vi "RVHR - File Selection.vi"(8 "error in":errorcluster) -> (0 "error out":errorcluster, 2 "cancelled?":bool caption="cancelled", 3 "RVHR path":path caption="selected path")   [LabVIEW 2024]
uses:
  Controls/Device_Type.ctl
  Controls/Language.ctl
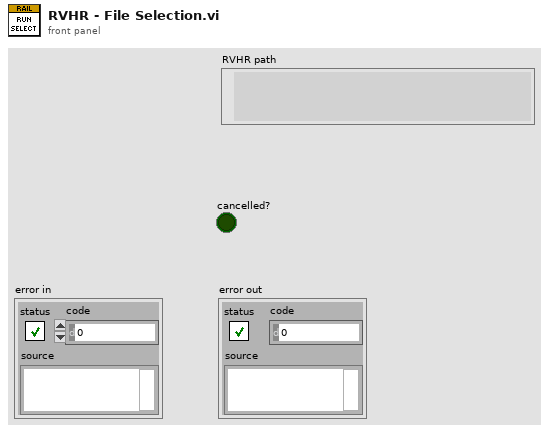
[diagram p1: front panel]
types:
  T1 = typedef "Device_Type.ctl" = enum16{"CAT", "Bi-CAT", "YRCA", "RCA", "RV-HR", "TV-HR"}
  T2 = typedef "Language.ctl" = enum16{"English", "Chinese", "German"}
  T3 = cluster{"Run Start":dbl, "Run End":dbl, "Date":timestamp}
  T4 = typedef "RVHR - Local Data.ctl" = cluster{"Main Filtered Data":dbl[][][], "Main Dist Data":dbl[], "Comp Filtered Data":dbl[][][], "Comp Dist Data":dbl[], "Image":u16, "Total Images":u16, "Main Test Cluster":T5, "Main Dates-Times":cluster{"Start Date":string, "Start Time":string, "Finish Time":string}, "Comp Test Cluster":T5, "Comp Dates-Times":cluster{"Start Date":string, "Start Time":string, "Finish Time":string}, "Comp Offset (mm)":i64, "XY Highlight Distance":dbl[], "Left Exc Info":T6[], "Right Exc Info":T6[], "Custom Start-Point":dbl, "UI Start-Distance":dbl, "UI End-Distance":dbl, "Distance Format":u8, "Language":T2, "Vision?":bool, "Left Image Folder":path, "Filename _L":string[], "Image Distances _L":dbl[], "Image Inc (km)":dbl, "Device Type":T1, "Panel Bounds":T7, "Panel Size":T8, "Version":string, "db Filepath":path, "Image Display Scale Factor":dbl}
  T5 = typedef "Test Cluster.ctl" = cluster{"Operator":string, "Description":string, "Line":string, "Start Position":dbl, "Run Length":dbl, "Sensor A Position":dbl, "Rail Side":bool, "Distance Direction":bool, "Path":path, "Sensor B Position":dbl, "Visible Chart Distance":dbl, "Company":string, "Ref Profile":string}
  T6 = typedef "Excluded Information.ctl" = cluster{"Start Dist":dbl, "End Dist":dbl, "Comments":string}
  T7 = typedef "LVRectTypeDef.ctl" = cluster{"Left":i16, "Top":i16, "Right":i16, "Bottom":i16}
  T8 = typedef "LVBoundsTypeDef.ctl" = cluster{"Width":u32, "Height":u32}
  T9 = typedef "Sum File Cluster (RCA).ctl" = cluster{"File Information":T10, "Run Description":T11, "Run Information":T12, "System Information":T13}
  T10 = typedef "File Information CLuster.ctl" = cluster{"Filename":path}
  T11 = typedef "Run Description.ctl" = cluster{"Description":string}
  T12 = typedef "Run information (YRCA).ctl" = cluster{"Operator":string, "Line":string, "Start Position":string, "End Position":string, "Run Length":string, "Direction":string, "Rail":string, "Run Graph Scale":u16, "Start Date":string, "Start Time":string, "Finish Time":string, "Company":string, "Ref Profile":string}
  T13 = typedef "System information (YRCA - Truncate).ctl" = cluster{"Sensor Calibration":string, "Integrator Time Constant":string, "Long Wavelength Filter":bool, "Tacho Pulses/Rev":string, "Wheel Diameter":string, "Sampling Distance":string, "Software Version":string, "Truncate Spectrum":bool}
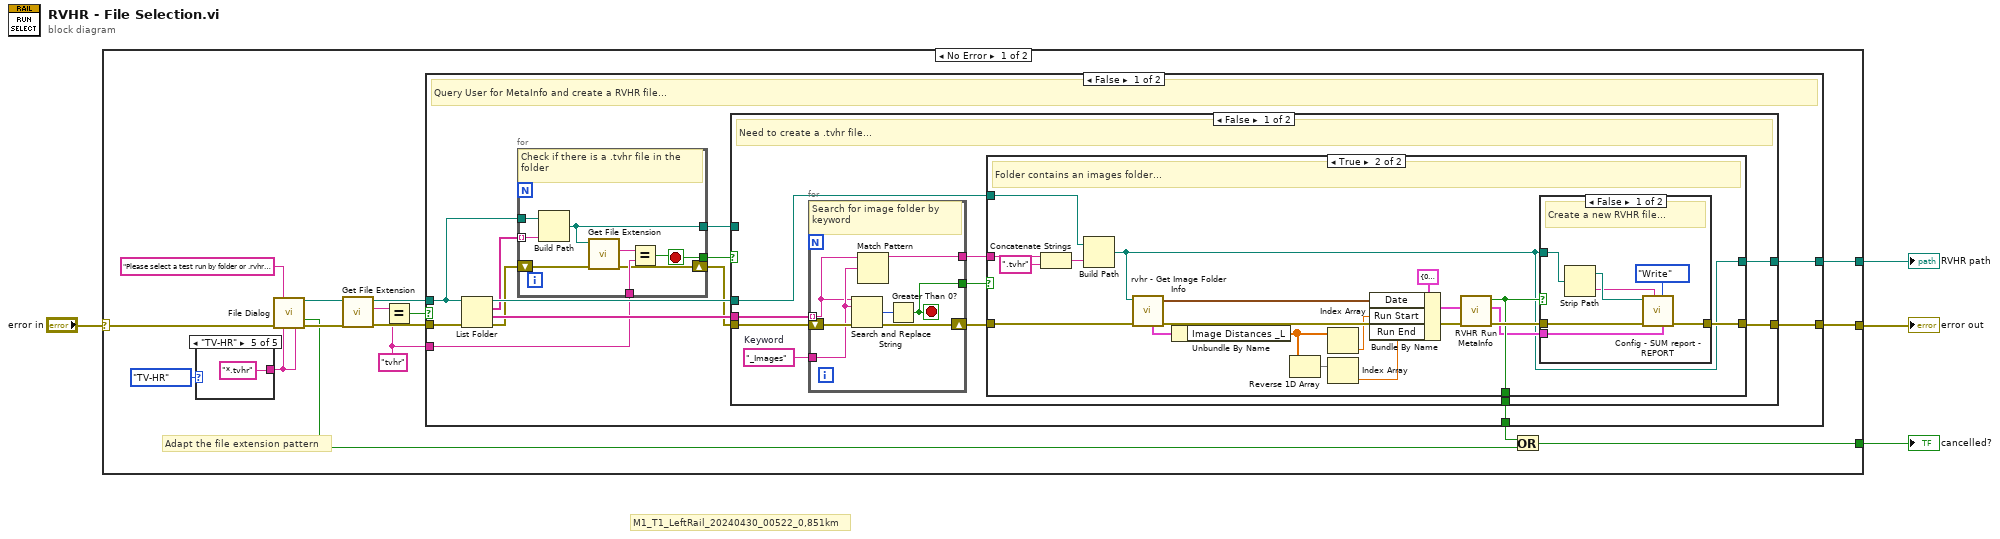
[diagram p0: block diagram]
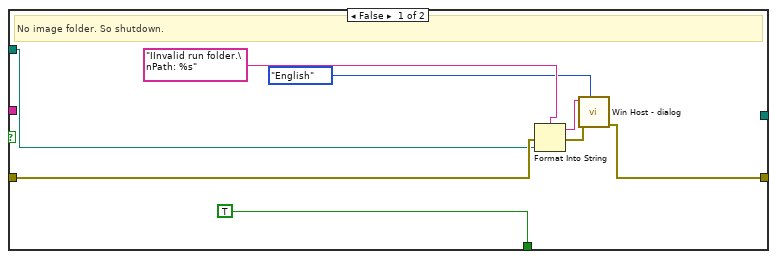
[diagram p2: hidden frame]
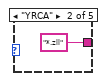
[diagram p7: hidden frame]
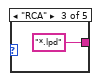
[diagram p8: hidden frame]
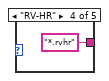
[diagram p9: hidden frame]
diagram:
  # "M1_T1_LeftRail_20240430_00522_0,851km"
  n1 = case shown="No Error" "error in" {
    selector: "error in" -> [w17 w102]
    tunnel: [w8 _] -> w2
    tunnel: [w9 w102] -> w1
    tunnel: [w6 _] -> w3
    frame No Error {
      w7 = "tvhr" ("y")
      # "Adapt the file extension pattern"
      n2 = case shown="\"TV-HR\"" Device_Type."TV-HR" ("Device Type") {
        tunnel: [_ "*.zll" ("pattern (all files)") "*.lpd" ("pattern (all files)") "*.rvhr" ("pattern (all files)") "*.tvhr" ("pattern (all files)")] -> w19
        frame "CAT", Default {
        }
        frame "YRCA" {
        }
        frame "RCA" {
        }
        frame "RV-HR" {
        }
        frame "TV-HR" {
        }
      }
      n3 = call "File Dialog"("prompt"="Please select a test run by folder or .rvhr file...", "error in"=w17, "pattern (all files)"=w19, "pattern label"=w19) -> ("selected path"=w15:path, "cancelled"=w14:bool, "error out"=w16:errorcluster)  [unwired: 8 in, 1 out]
      n4 = call <vilib>:"Get File Extension.vi"("error in (no error)"=w16, "file"=w15) -> ("error out"=w11:errorcluster, "lowercase file extension"=w13:string, "dup file"=w10:path)  [unwired: 5 in, 2 out]
      n5 = Equal?(x=w13, y=w7) -> (x = y?=w12:bool)
      n6 = case shown="False" w12 {
        tunnel: w11 -> [w30 w97]
        tunnel: w10 -> [w25 w96]
        tunnel: [w33 w97] -> w9
        tunnel: [w32 w96] -> w8
        tunnel: w7 -> [w24 _]
        tunnel: [w31 _] -> w5
        frame False {
          # "Query User for MetaInfo and create a RVHR file..."
          n7 = List Folder(path=w25, error in=w30) -> (path out=w28:path, filenames=w27:string[], folder names=w29:string[], error out=w26:errorcluster)  [unwired: 2 in]
          n8 = for {
            tunnel: w27 -> [w40] mode=indexing
            shift-right: [w36] -> w22
            shift-left: w26 -> [w41]
            tunnel: w25 -> [w39]
            tunnel: w24 -> [w37]
            tunnel: [w35] -> w23
            tunnel: [w34] -> w21
            stop <- w35 stop-if-true
            # "Check if there is a .tvhr file in the folder"
            n9 = Build Path(base path=w39, name or relative path=w40) -> (appended path=w34:path)
            n10 = call <vilib>:"Get File Extension.vi"("error in (no error)"=w41, "file"=w34) -> ("error out"=w36:errorcluster, "lowercase file extension"=w38:string)  [unwired: 5 in, 3 out]
            n11 = Equal?(x=w38, y=w37) -> (x = y?=w35:bool)
          }
          n12 = case shown="False" w23 {
            tunnel: [w51 w95] -> w33
            tunnel: [w50 w94] -> w32
            tunnel: [w49 _] -> w31
            tunnel: w22 -> [w48 w95]
            tunnel: w29 -> [w47 _]
            tunnel: w28 -> [w44 _]
            tunnel: w21 -> [_ w94]
            frame False {
              w46 = "_Images"  # Keyword
              # "Need to create a .tvhr file..."
              n13 = for {
                tunnel: w46 -> [w55]
                shift-right: [w56] -> w43
                shift-left: w48 -> [w58]
                tunnel: w47 -> [w54] mode=indexing
                tunnel: [w53] -> w45
                tunnel: [w52] -> w42
                stop <- w52 stop-if-true
                # "Search for image folder by keyword"
                n14 = Search and Replace String(input string=w54, search string=w55, error in=w58) -> (number of replacements=w57:i32, error out=w56:errorcluster)  [unwired: 5 in, 2 out]
                n15 = Match Pattern(string=w54, regular expression=w55) -> (before substring=w53:string)  [unwired: 1 in, 3 out]
                n16 = Greater Than 0?(x=w57) -> (x > 0?=w52:bool)
              }
              n17 = case shown="True" w42 {
                tunnel: [w62 w83] -> w51
                tunnel: [_ w75] -> w50
                tunnel: [TRUE ("Cancel?") w82] -> w49
                tunnel: w43 -> [w61 w77]
                tunnel: w45 -> [_ w79]
                tunnel: w44 -> [w59 w78]
                frame False {
                  # "No image folder. So shutdown."
                  n18 = Format Into String(format string="IInvalid run folder.\nPath: %s" ("Message"), error in=w61, w59) -> (resulting string=w65:string, error out=w63:errorcluster)  [unwired: 1 in]
                  n19 = call "Win Host - dialog.vi"("Language"=Language."English", "error in (no error)"=w63, "Message"=w65) -> ("error out"=w62:errorcluster)  [unwired: 7 in, 1 out]
                }
                frame True {
                  # "Folder contains an images folder..."
                  n20 = Concatenate Strings(w79, ".tvhr" ("string")) -> (w85:string)
                  n21 = Build Path(base path=w78, name or relative path=w85) -> (appended path=w75:path)
                  n22 = call "rvhr - Get Image Folder Info.vi"("error in (no error)"=w77, "selected path"=w75) -> ("error out"=w76:errorcluster, "Time Stamp"=w67:timestamp, "Local Data out"=w72:T4)  [unwired: 7 in]
                  n23 = Unbundle By Name(w72) -> ("Image Distances _L"=w68:dbl[])
                  n24 = Reverse 1D Array(array=w68) -> (reversed array=w69:dbl[])
                  n25 = Index Array(array=w68) -> (element=w71:dbl)  [unwired: 1 in]
                  n26 = Index Array(array=w69) -> (element=w70:dbl)  [unwired: 1 in]
                  n27 = Bundle By Name(cluster=T3 {"Run Start"=0.0, "Run End"=0.0, "Date"=timestamp(0 s since 1904-01-01)} ("Run Info"), "Date"=w67, "Run Start"=w71, "Run End"=w70) -> (w73:T3)
                  n28 = call "RVHR Run MetaInfo.vi"("error in (no error)"=w76, "Run Info"=w73) -> ("error out"=w84:errorcluster, "RVHR Info File"=w81:T9, "Cancel?"=w82:bool)  [unwired: 7 in]
                  n29 = case shown="False" w82 {
                    tunnel: w84 -> [w91 w93]
                    tunnel: [w90 w93] -> w83
                    tunnel: w75 -> [w89 _]
                    tunnel: w81 -> [w86 _]
                    frame False {
                      # "Create a new RVHR file..."
                      n30 = Strip Path(path=w89) -> (stripped path=w88:path, name=w87:string)
                      n31 = call "Config - SUM report - REPORT.vi"("RVHR Cluster In"=w86, ".ini Controller"=enum16{"Read", "Write"}."Write", ".ini filename"=w87, "error in (no error)"=w91, "Directory Path"=w88) -> ("error out"=w90:errorcluster)  [unwired: 4 in, 2 out]
                    }
                    frame True {
                      # "Cancelled..."
                    }
                  }
                }
              }
            }
            frame True {
              # "Already one exists..."
            }
          }
        }
        frame True {
          # "Already has a .rvhr file. Do nothing..."
        }
      }
      n32 = Or(x=w5, y=w14) -> (x .or. y?=w6:bool)
    }
    frame Error {
    }
  }
  "RVHR path" <- w2
  "error out" <- w1
  "cancelled?" <- w3
